vi "Apply Audiogram Compensation.vi"(0 "Audiogram File":path=path "C:/Users/Ken/Desktop/Mouse Audiogram.txt", 7 "Noise In":dbl[](array[numeric]), 9 "Sampling Rate (Hz)":dbl, 11 "error in (no error)":errorcluster) -> (6 "Compensated Noise":dbl[](graph), 10 "Ref Adjust":dbl, 14 "audiogram min (dB SPL)":dbl, 15 "error out":errorcluster)   [LabVIEW 2020]
uses:
  epl-vi-lib/Utility VIs/Math VIs/LinSpace (x0-dx-npts).vi
  epl-vi-lib/Utility VIs/Math VIs/FFT x(t) to dB,Degrees (1D).vi
  epl-vi-lib/Utility VIs/Math VIs/dB to Linear (1D).vi
  epl-vi-lib/Utility VIs/Math VIs/Linear to dB (array).vi
  epl-vi-lib/Utility VIs/Math VIs/Linear to dB (scalar).vi
panel:
  out "Comp Mag Spec":cluster{dbl[], dbl[]}(graph)
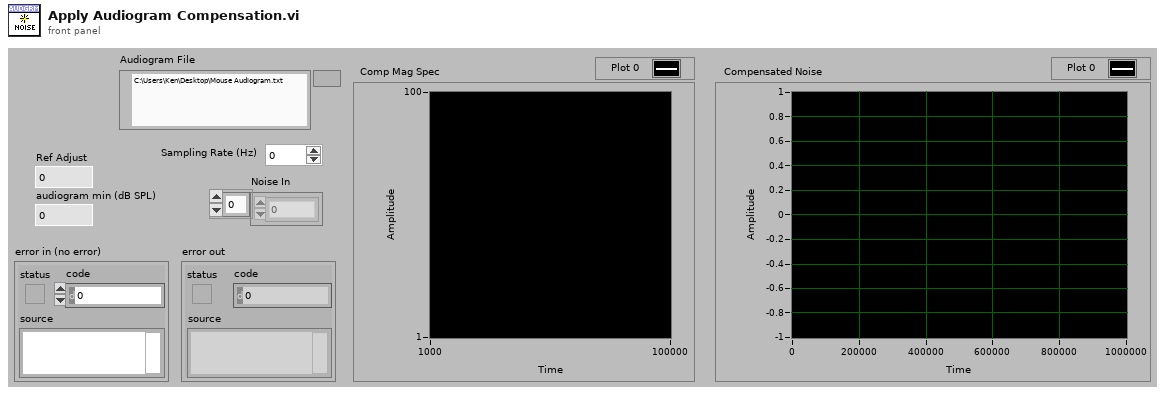
[diagram p1: front panel]
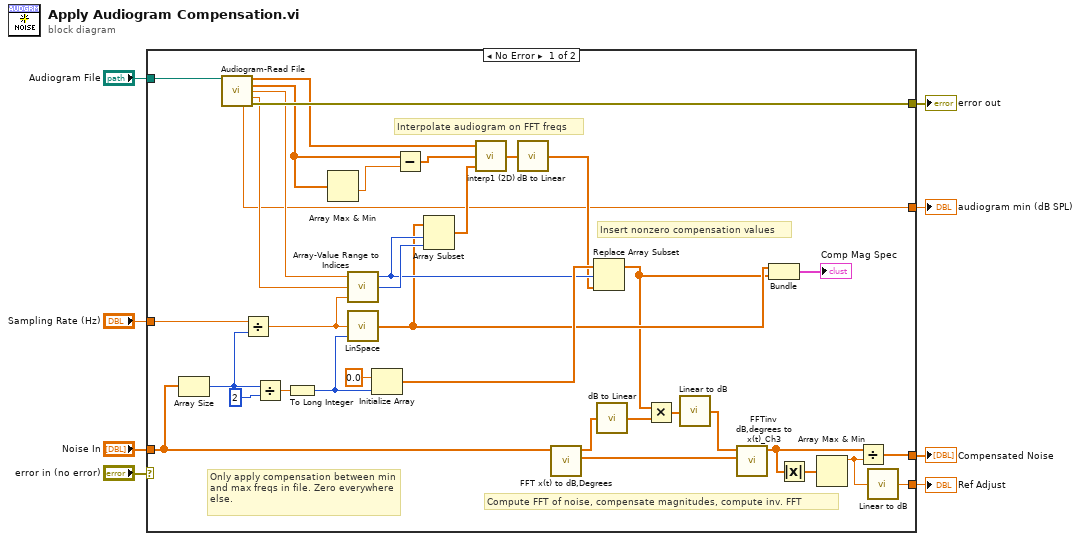
[diagram p0: block diagram]
diagram:
  n1 = case shown="No Error" "error in (no error)" {
    selector: "error in (no error)" -> [_ w45]
    tunnel: [w42 w45] -> w7
    tunnel: "Audiogram File" -> [w43 _]
    tunnel: [w44 _] -> w5
    tunnel: "Noise In" -> [w20 _]
    tunnel: "Sampling Rate (Hz)" -> [w18 _]
    tunnel: [w11 _] -> w2
    tunnel: [w9 _] -> w1
    frame No Error {
      # "Compute FFT of noise, compensate magnitudes, compute inv. FFT"
      # "Insert nonzero compensation values"
      # "Interpolate audiogram on FFT freqs"
      # "Only apply compensation between min and max freqs in file. Zero everywhere else."
      n2 = Array Size(array=w20) -> (size(s)=w21:i32)
      n3 = call "Audiogram-Read File.vi"("Audiogram File"=w43) -> ("Freq (Hz)"=w17:dbl[], "Magnitude (dB)"=w14:dbl[], "MinFreq (Hz)"=w16:dbl, "MaxFreq (Hz)"=w15:dbl, "Min Threshold (dB SPL)"=w9:dbl, "error out"=w42:errorcluster)  [unwired: 8 in, 1 out]
      n4 = Divide(x=w18, y=w21) -> (x/y=w41:dbl)
      n5 = Divide(x=w21, y=2) -> (x/y=w38:dbl)
      n6 = To Long Integer(number=w38) -> (32bit integer=w36:i32)
      n7 = Array Max & Min(array=w14) -> (min value=w10:dbl)  [unwired: 3 out]
      n8 = call "Array-Value Range to Indices.vi"("dx"=w41, "Xmax"=w15, "Xmin"=w16) -> ("Length"=w40:i32, "Offset"=w33:i32)  [unwired: 1 in]
      n9 = call-poly "LinSpace.vi"("npts"=w36, "dx"=w41) -> ("Array"=w31:dbl[])  [unwired: 2 in, 1 out]
      n10 = Initialize Array(0.0 ("element"), w36) -> (w34:dbl[])
      n11 = Subtract(x=w14, y=w10) -> (x-y=w13:dbl[])
      n12 = Array Subset(array=w31, index=w33, length=w40) -> (w39:dbl[])
      n13 = call "interp1 (2D).vi"("X"=w17, "Y"=w13, "U"=w39) -> ("V"=w32:dbl[])  [unwired: 2 in]
      n14 = call-poly "dB to Linear.vi"("dB"=w32) -> ("linear"=w24:dbl[])
      n15 = call-poly "FFT x(t) to dB,Degrees.vi"("X"=w20) -> ("+Freq Phase of FFT (degrees)"=w29:dbl[], "+Freq. Mag of FFT (dB rms)"=w26:dbl[])  [unwired: 8 in, 1 out]
      n16 = Replace Array Subset(array=w34, new element=w24, index=w33) -> (w19:dbl[])
      n17 = call-poly "dB to Linear.vi"("dB"=w26) -> ("linear"=w25:dbl[])
      n18 = Multiply(x=w19, y=w25) -> (x*y=w23:dbl[])
      n19 = call-poly "Linear to dB.vi"("linear"=w23) -> ("dB"=w22:dbl[])
      n20 = call "FFTinv dB,degrees to x(t)_Ch3.vi"("+Freq Phase of FFT (degrees)"=w29, "+Freq. Mag of FFT (rms dB)"=w22) -> ("X(t)"=w27:dbl[])  [unwired: 8 in, 1 out]
      n21 = Bundle("Array"=w31, w19) -> (→"Comp Mag Spec":cluster{"Array":dbl[], dbl[]})  [unwired: 1 in]
      n22 = Absolute Value(x=w27) -> (abs(x)=w28:dbl[])
      n23 = Array Max & Min(array=w28) -> (max value=w12:dbl)  [unwired: 3 out]
      n24 = Divide(x=w27, y=w12) -> (x/y=w44:dbl[])
      n25 = call-poly "Linear to dB.vi"("Linear"=w12) -> ("dB"=w11:dbl)
    }
    frame Error {
    }
  }
  "error out" <- w7
  "Compensated Noise" <- w5
  "Ref Adjust" <- w2
  "audiogram min (dB SPL)" <- w1
